vi "OpenVariant Tree Example.vi"() -> ()   [LabVIEW 2020]
uses:
  _built_ppls/OpenVariant.lvlibp
panel:
  out "KVP":variant
  out "Variant":variant
  in  "Tree":string(tree)
  out "Variant Tree":variant
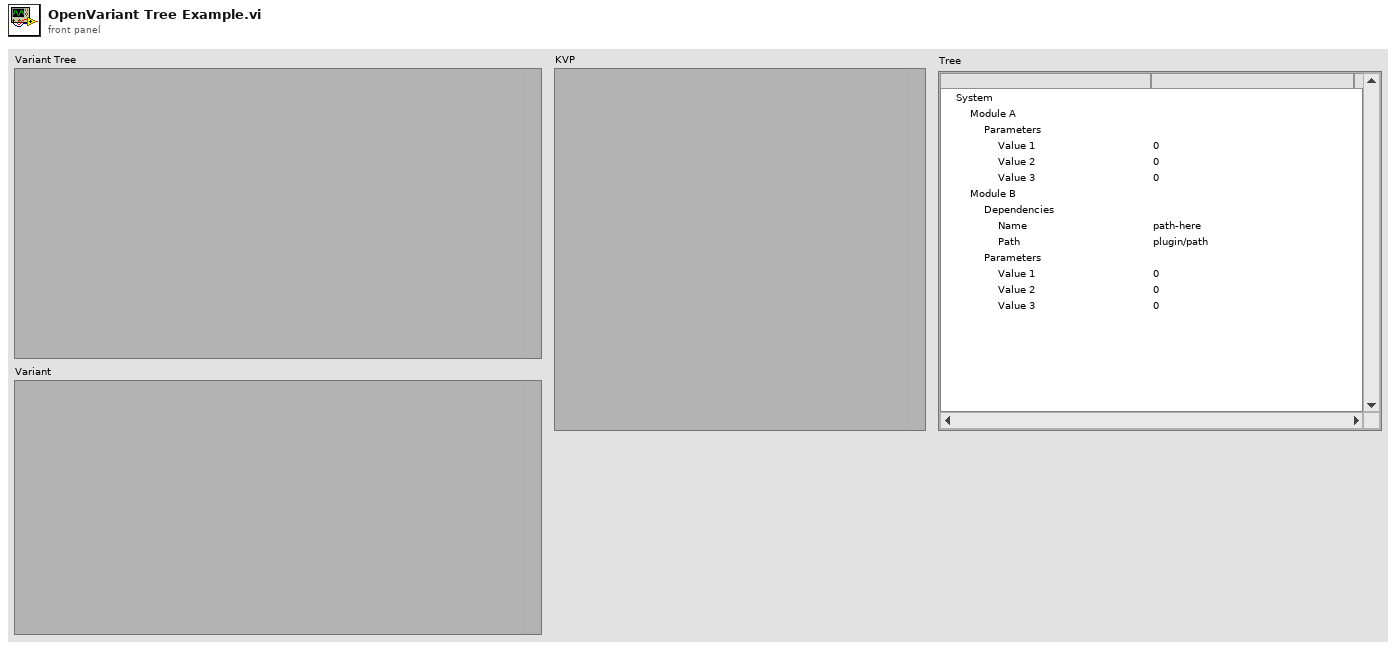
[diagram p1: front panel]
types:
  T1 = cluster{"Module A":cluster{"Parameters":cluster{"Value 1":dbl, "Value 2":dbl, "Value 3":dbl}}, "Module B":cluster{"Parameters":cluster{"Value 1":dbl, "Value 2":dbl, "Value 3":dbl}, "Dependencies":cluster{"Name":string, "Path":path}}}
  T2 = cluster{"Left Cell String":string, "Child Text":string[], "Child Tag":string, "Item Indent":i32, "Child Only?":bool, "Glyph Index":i32}[]
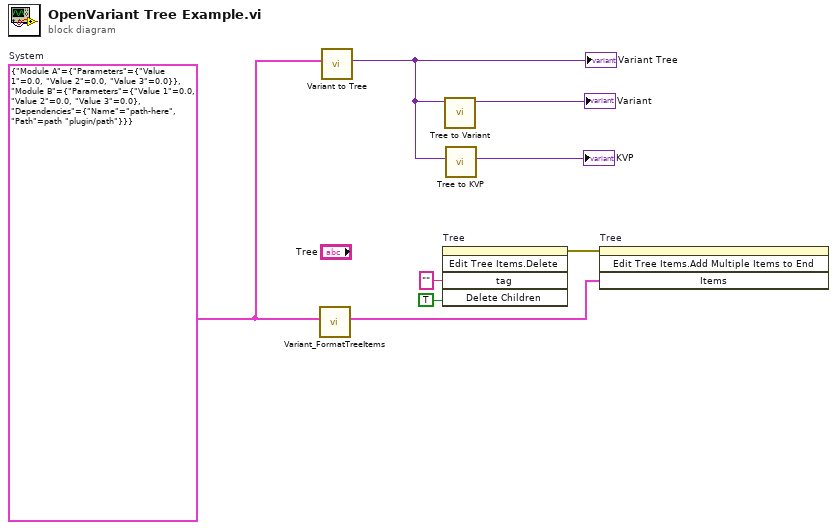
[diagram p0: block diagram]
diagram:
  w4 = T1 {"Module A"={"Parameters"={"Value 1"=0.0, "Value 2"=0.0, "Value 3"=0.0}}, "Module B"={"Parameters"={"Value 1"=0.0, "Value 2"=0.0, "Value 3"=0.0}, "Dependencies"={"Name"="path-here", "Path"=path "plugin/path"}}}  # System
  n1 = call "Variant_FormatTreeItems.vi"("Variant"=w4) -> ("Tree Items"=w8:T2)  [unwired: 10 in]
  n2 = call "Variant to Tree.vi"("Variant"=w4) -> ("Variant Tree"=w2:variant)  [unwired: 10 in]
  "Variant Tree" <- w2
  n3 = invoke on="Tree" class="Tree (strict)" method="Edit Tree Items.Delete"("tag"="" ("Tag"), "Delete Children"=TRUE ("Delete Children?")) -> (error out=w7:errorcluster)  [unwired: 3 in, 4 out]
  n4 = call "Tree to Variant.vi"("Variant Tree"=w2) -> ("Variant"=→"Variant":variant)  [unwired: 10 in]
  n5 = call "Tree to KVP.vi"("Variant Tree"=w2) -> ("KVP"=→"KVP":variant)  [unwired: 10 in]
  n6 = invoke on="Tree" class="Tree (strict)" method="Edit Tree Items.Add Multiple Items to End"(error in=w7, "Items"=w8) -> ()  [unwired: 2 in, 4 out]
